vi "Transpose Export Error Code.vi"(8 "error in (no error)":errorcluster, 11 "Test Report":refnum<class "Test Report.lvclass">) -> (0 "error out":errorcluster, 3 "Test Report out":refnum<class "Test Report.lvclass">)   [LabVIEW 2013, in "Caraya.lvlib" / "Test Report.lvclass"]
uses:
  Test Report.lvclass
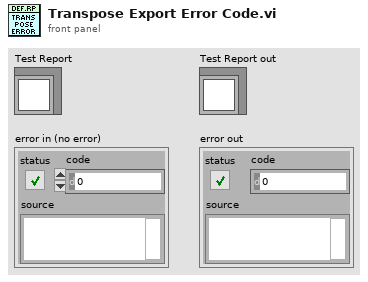
[diagram p1: front panel]
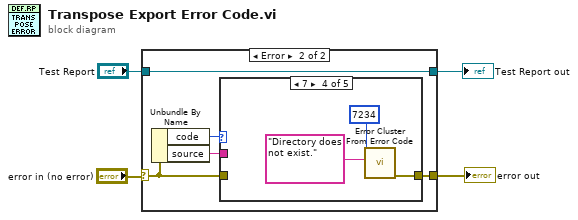
[diagram p0: block diagram]
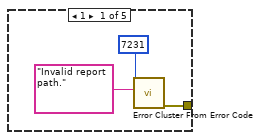
[diagram p3: hidden frame]
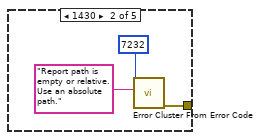
[diagram p4: hidden frame]
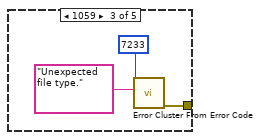
[diagram p5: hidden frame]
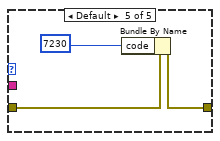
[diagram p6: hidden frame]
diagram:
  n1 = case shown="Error" "error in (no error)" {
    selector: "error in (no error)" -> [w6 w10]
    tunnel: [w6 w11] -> w1
    tunnel: "Test Report" -> [w5 w7]
    tunnel: [w5 w7] -> w4
    frame No Error {
    }
    frame Error {
      n2 = Unbundle By Name(w10) -> ("code"=w9:i32, "source"=w8:string)
      n3 = case shown="7" w9 {
        tunnel: w10 -> [_ _ _ _ w26]
        tunnel: [w13 w16 w19 w22 w25] -> w11
        tunnel: w8 -> [_ _ _ _ _]
        frame 1 {
          n4 = call <vilib>:"Error Cluster From Error Code.vi"("error message (\"\")"="Invalid report path." ("error message (\"\")"), "error code (0)"=7231) -> ("error out"=w13:errorcluster)  [unwired: 7 in]
        }
        frame 1430 {
          n5 = call <vilib>:"Error Cluster From Error Code.vi"("error message (\"\")"="Report path is empty or relative. Use an absolute path." ("error message (\"\")"), "error code (0)"=7232) -> ("error out"=w16:errorcluster)  [unwired: 7 in]
        }
        frame 1059 {
          n6 = call <vilib>:"Error Cluster From Error Code.vi"("error message (\"\")"="Unexpected file type." ("error message (\"\")"), "error code (0)"=7233) -> ("error out"=w19:errorcluster)  [unwired: 7 in]
        }
        frame 7 {
          n7 = call <vilib>:"Error Cluster From Error Code.vi"("error message (\"\")"="Directory does not exist." ("error message (\"\")"), "error code (0)"=7234) -> ("error out"=w22:errorcluster)  [unwired: 7 in]
        }
        frame Default {
          n8 = Bundle By Name(cluster=w26, "code"=7230 ("error code (0)")) -> (w25:errorcluster)
        }
      }
    }
  }
  "Test Report out" <- w4
  "error out" <- w1
